vi "create ROIs GUI.vi"(9 "Mask high value (default 255)":sgl=255.0, 11 "TIFF path":path) -> (0 "error out":errorcluster, 3 "ROI mask image":T1)   [LabVIEW 2025]
uses:
  <vilib>/vision/Image Controls.llb/IMAQ Image.ctl
  <vilib>/vision/NI_Vision_Development_Module.lvlib
panel:
  out "Image 3":T1(plugin-control)
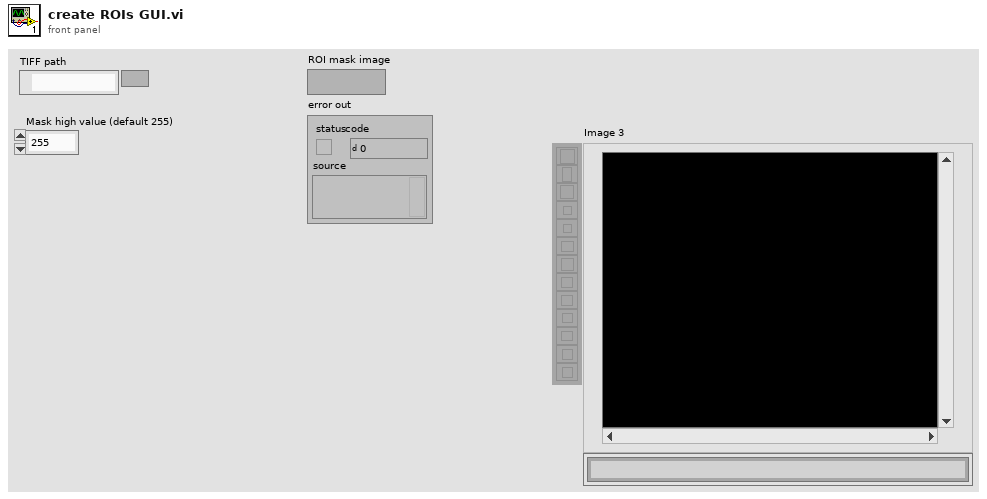
[diagram p1: front panel]
types:
  T1 = typedef "IMAQ Image.ctl" = refnum<image>
  T2 = typedef "Image Type" = u32
  T3 = typedef "ROI Descriptor" = cluster{"Global Rectangle":i32[], "Contours":cluster{"ID":enum32{"External", "Internal"}, "Type":u32, "Coordinates":i32[]}[]}
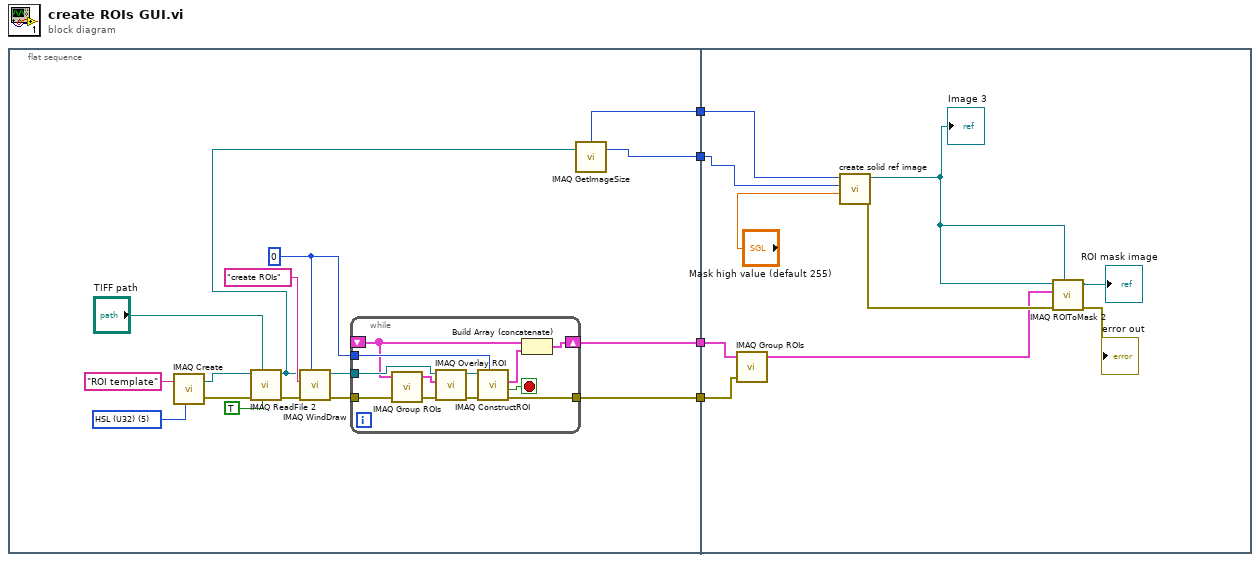
[diagram p0: block diagram]
diagram:
  n1 = flat-sequence {
    tunnel: [w11] -> w4
    tunnel: [w10] -> w3
    tunnel: [w7] -> w2
    tunnel: [w8] -> w1
    tunnel: w4 -> [w42]
    tunnel: w3 -> [w41]
    tunnel: w2 -> [w34]
    tunnel: w1 -> [w35]
    frame #0 {
      w15 = 0 ("Window Number (0...15)")
      w18 = T2 5 items=["Grayscale (U8)", "Grayscale (I16)", "Grayscale (SGL)", "Complex (CSG)", "RGB (U32)", "HSL (U32)", "RGB (U64)", "Grayscale (U16)"] ("Image Type")
      n2 = call "IMAQ Create"("Image Name"="ROI template", "Image Type"=w18) -> ("New Image"=w5:T1, "error out"=w14:errorcluster)  [unwired: 3 in]
      n3 = call "IMAQ ReadFile 2"("Use File Path Image Type"=TRUE, "File Path"="TIFF path", "error in (no error)"=w14, "Image"=w5) -> ("error out"=w19:errorcluster, "Image Out"=w6:T1)  [unwired: 3 in, 3 out]
      n4 = call "IMAQ WindDraw"("Window Number (0...15)"=w15, "error in (no error)"=w19, "Title"="create ROIs", "Image"=w6) -> ("error out"=w13:errorcluster, "Image Out (duplicate)"=w9:T1)  [unwired: 6 in]
      n5 = while {
        tunnel: w9 -> [w29]
        tunnel: w15 -> [w32]
        shift-right: [w24] -> w11
        shift-left: _ -> [w25]
        tunnel: [w30] -> w10
        tunnel: w13 -> [w21]
        stop <- w31 stop-if-true
        n6 = call "IMAQ Group ROIs"("error in (no error)"=w21, "ROI Descriptors"=w25) -> ("error out"=w22:errorcluster, "ROI Descriptor out"=w27:T3)  [unwired: 2 in]
        n7 = call "IMAQ Overlay ROI"("error in (no error)"=w22, "ROI Descriptor"=w27, "Image"=w29) -> ("error out"=w23:errorcluster, "Image Out"=w28:T1)  [unwired: 7 in]
        n8 = call "IMAQ ConstructROI"("Window Number (-1...15)"=w32, "error in (no error)"=w23, "Image"=w28) -> ("error out"=w30:errorcluster, "Cancel"=w31:bool, "ROI Descriptor Out"=w26:T3)  [unwired: 5 in, 1 out]
        n9 = Build Array (concatenate)(w25, w26) -> (w24:T3[])
      }
      n10 = call "IMAQ GetImageSize"("Image"=w6) -> ("Y Resolution"=w7:i32, "X Resolution"=w8:i32)  [unwired: 3 in, 1 out]
    }
    frame #1 {
      n11 = call "IMAQ Group ROIs"("error in (no error)"=w41, "ROI Descriptors"=w42) -> ("ROI Descriptor out"=w36:T3)  [unwired: 2 in, 1 out]
      n12 = call "create solid ref image.vi"("Pixel Value (default 255)"="Mask high value (default 255)", "Y resolution"=w34, "X resolution"=w35) -> ("error out"=w38:errorcluster, "solid image"=w33:T1)  [unwired: 7 in]
      "Image 3" <- w33
      n13 = call "IMAQ ROIToMask 2"("Image Model"=w33, "error in (no error)"=w38, "ROI Descriptor"=w36, "Image"=w33) -> ("error out"=→"error out":errorcluster, "Image Out"=→"ROI mask image":T1)  [unwired: 5 in, 1 out]
    }
  }
